vi "Rohwerte skalieren.vi"(1 "GasValue":sgl[](array[numeric]), 2 "Messwert umschalten":bool, 12 "CAL-Daten":T1={"O2 Null"=0.0, "O2 Steil"=[1.0, 1.0, 1.0, 1.0]}) -> (4 "Messwerte":sgl[](array[numeric]), 6 "Rohwerte":sgl[](array[numeric]), 8 "Rohwerte LIN":sgl[](array[numeric]))   [LabVIEW 2020, in "ABB-EL3000.lvlib" / "PMA.lvlib" / "Kalibrieren.lvlib"]
uses:
  Kalibrieren.lvlib
  Allgemeine VI/CAL-Daten PMA.ctl
  Linearisierung V2/Linearisierung v2.lvlib
  PMA.lvlib
  Allgemeine VI/Allgemeine VI.lvlib
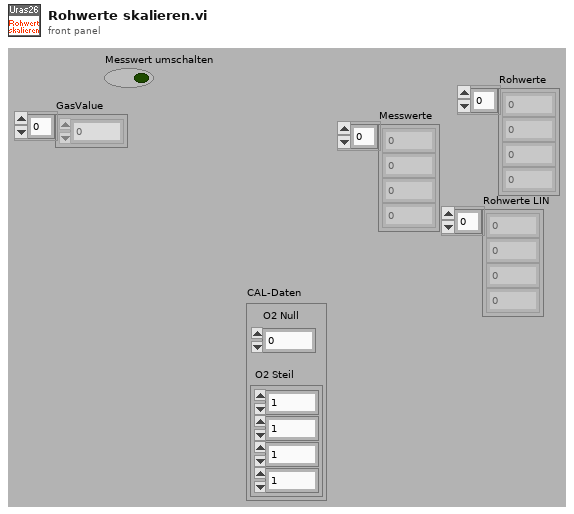
[diagram p1: front panel]
types:
  T1 = typedef "ABB-EL3000.lvlib/Allgemeine VI.lvlib/CAL-Daten PMA.ctl" = cluster{"O2 Null":sgl, "O2 Steil":sgl[]}
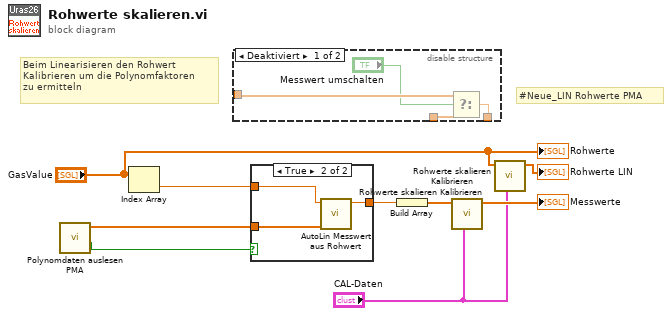
[diagram p0: block diagram]
diagram:
  # "#Neue_LIN Rohwerte PMA"
  # "Beim Linearisieren den Rohwert \nKalibrieren um die Polynomfaktoren \nzu ermitteln"
  n1 = call "Polynomdaten auslesen PMA.vi"() -> ("Aktiv"=w4:bool, "Teil-Array"=w5:dbl[])  [unwired: 9 in, 1 out]
  n2 = Index Array(array="GasValue") -> (element=w8:sgl)  [unwired: 1 in]
  n3 = disable-structure shown="Deaktiviert" {
    disable-tunnel: _ -> [w13 _]
    disable-tunnel: _ -> [w12 _]
    disable-tunnel: [w11 _] -> _
    frame Disabled {
      n4 = Select(t=w13, s="Messwert umschalten", f=w12) -> (s? t:f=w11:dbl)
    }
    frame Enabled {
    }
  }
  n5 = case shown="True" w4 {
    tunnel: w8 -> [w14 w17]
    tunnel: w5 -> [_ w15]
    tunnel: [w14 w16] -> w7
    frame False {
    }
    frame True {
      n6 = call "AutoLin Messwert aus Rohwert.vi"("Polynomkoeff."=w15, "Rohwert (ppm)"=w17) -> ("Messwert (ppm) linearisiert"=w16:dbl)  [unwired: 9 in]
    }
  }
  n7 = Build Array(w7) -> (w6:dbl[])
  n8 = call "Rohwerte skalieren Kalibrieren.vi"("CAL-Daten"="CAL-Daten", "GasValue"=w6) -> ("Kalibrierte Rohwerte"=→"Messwerte":sgl[])  [unwired: 9 in]
  n9 = call "Rohwerte skalieren Kalibrieren.vi"("CAL-Daten"="CAL-Daten", "GasValue"="GasValue") -> ("Kalibrierte Rohwerte"=→"Rohwerte LIN":sgl[])  [unwired: 9 in]
  "Rohwerte" <- "GasValue"
